vi "Measurement UI.vi"() -> ()   [LabVIEW 2021, in "Line Transient_Channel Ganging UI.lvlib"]
uses:
  Line Transient_Channel Ganging UI.lvlib
panel:
  in  "MeasGraphs":T1(tab)
  out "InputVoltageV/STimeGraph":waveform(dbl)(graph) caption="Load Transient"
  out "OutputVoltageV/STimeGraph":waveform(dbl)(graph) caption="Load Transient"
  in  "Source Voltage v/s Time":string="SOURCE VOLTAGE vs TIME"
  in  "Output Voltage v/s Time":string="LOAD VOLTAGE vs TIME"
  out "InputVoltageV/STimeGraphScope":waveform(dbl)(graph) caption="Load Transient"
  in  "ScopeSource Voltage v/s Time":string="SOURCE VOLTAGE vs TIME"
  out "OutputVoltageV/STimeScope":waveform(dbl)(graph) caption="Load Transient"
  in  "ScopeOutput Voltage v/s Time":string="LOAD VOLTAGE vs TIME"
  out "Scope dt":dbl
  out "Source voltages":dbl[](array[numeric])
  out "Scope amplitudes":dbl[](array[numeric])
  out "Load voltages":dbl[](array[numeric])
  out "Smu dt":dbl
  in  "Load current pole-zero ratio":dbl=0.3
  in  "Load current compensation frequency":dbl=180000.0
  in  "Load current gain bandwidth":dbl=14000.0
  in  "Source voltage pole-zero ratio":dbl=2.0
  in  "Source voltage compensation frequency":dbl=3530.0
  in  "Source voltage gain bandwidth":dbl=2000.0
  in  "Load slave resource names":string[](array[string])
  in  "Load master resource name":string
  in  "Source slave resource names":string[](array[string])
  in  "Source master resource name":string
  in  "Scope resource name":string
  in  "MeasConfigurations":T2(tab)=enum."Source Config"
  in  "Nominal output voltage":dbl=1.0 caption="NOMINAL OUTPUT VOLTAGE" format="%.3pV"
  in  "DUT setup time":dbl=1.0 caption="DUT SETUP TIME" format="%.3ps"
  in  "Source pulse duration":dbl=0.001 caption="PULSE DURATION" format="%.3ps"
  in  "Source time delay 1":dbl=0.001 caption="TIME DELAY 1" format="%.3ps"
  in  "Source time delay 2":dbl=0.001 caption="TIME DELAY 2" format="%.3ps"
  in  "Source voltage level 2":dbl=20.0 caption="VOLTAGE LEVEL 2" format="%#_6pV"
  in  "Source voltage falling slew rate":dbl=6000.0 caption="VOLTAGE FALLING SLEW RATE" format="%#_6pV/s"
  in  "Source voltage rising slew rate":dbl=6000.0 caption="VOLTAGE RISING SLEW RATE" format="%#_6pV/s"
  in  "PPSSlaveResourceNames":refnum<k15>[](array[refnum]) caption="SLAVE RESOURCE NAMES"
  in  "PPSMasterResourceName":refnum<k15> caption="MASTER RESOURCE NAME"
  in  "Source transient response":i32(ring)=1038 caption="TRANSIENT RESPONSE" items=["Slow"=1041, "Normal"=1038, "Fast"=1039, "Custom"=1042]
  in  "Source sense":i32(ring)=1009 caption="SENSE" items=["Local"=1008, "Remote"=1009]
  in  "Source voltage level range":dbl=20.0 caption="VOLTAGE LEVEL RANGE" format="%#_6pV"
  in  "Source voltage level 1":dbl=12.0 caption="VOLTAGE LEVEL 1" format="%#_6pV"
  in  "Source current limit high":dbl=25.0 caption="CURRENT LIMIT/LIMIT HIGH" format="%#_6pA"
  in  "Source current limit range":dbl=25.0 caption="CURRENT LIMIT RANGE" format="%#_6pA"
  in  "Source limit symmetry":enum32{"Symmetric", "Asymmetric"}(ring)=enum."Asymmetric" caption="LIMIT SYMMETRY"
  in  "Source current limit low":dbl=-0.6 caption="CURRENT LIMIT LOW" format="%#_6pA"
  in  "Source system configuration":enum32{"Series", "Parallel"}(ring)=enum."Parallel" caption="SYSTEM CONFIG"
  in  "Source compliance":string="Compliance"
  in  "Source sourceadapt":string="SourceAdapt"
  in  "Source Custom Transient Response":bool
  in  "Source sample rate":dbl=1800000.0 caption="SAMPLE RATE" format="%#_6pS/s"
  in  "Load current level":dbl=1.0 caption="CURRENT LEVEL" format="%#_6pA"
  in  "Load sourceadapt":string="SourceAdapt"
  in  "Load compliance":string="Compliance"
  in  "Load system configuration":enum32{"Series", "Parallel"}(ring)=enum."Parallel" caption="SYSTEM CONFIG"
  in  "Load voltage limit low":dbl caption="VOLTAGE  LIMIT LOW" format="%#_6pV"
  in  "Load limit symmetry":enum32{"Symmetric", "Asymmetric"}(ring) caption="LIMIT SYMMETRY"
  in  "Load voltage limit range":dbl=6.0 caption="VOLTAGE LIMIT RANGE" format="%#_6pV"
  in  "Load voltage limit high":dbl=inf caption="VOLTAGE LIMIT/LIMIT HIGH" format="%#_6p"
  in  "Load current level range":dbl=80.0 caption="CURRENT LEVEL RANGE" format="%#_6pA"
  in  "Load sense":i32(ring)=1009 caption="SENSE" items=["Local"=1008, "Remote"=1009]
  in  "Load transient response":i32(ring)=1038 caption="TRANSIENT RESPONSE" items=["Slow"=1041, "Normal"=1038, "Fast"=1039, "Custom"=1042]
  in  "LoadSlaveResourceNames":refnum<k15>[](array[refnum]) caption="SLAVE RESOURCE NAMES"
  in  "LoadMasterResourceName":refnum<k15> caption="MASTER RESOURCE NAME"
  in  "Load Custom Transient Response":bool
  in  "Scope vertical range":dbl=10.0 caption="VERTICAL RANGE"
  out "Scope status":string="Scope is enabled"
  in  "Scope enable/disable":bool caption="Scope Enable/Disable"
  in  "SCOPEResourceName":refnum<k15> caption="RESOURCE NAME"
  in  "Scope probe attenuation":dbl=1.0 caption="PROBE ATTENUATION"
  in  "Scope sample rate":dbl=1800000.0 caption="SAMPLE RATE" format="%#_6pHz"
  in  "Scope output channel name":string="0" caption="OUTPUT CHANNEL NAME"
  in  "Scope vertical coupling":enum32{"AC", "DC"}(ring)=enum."DC" caption="VERTICAL COUPLING"
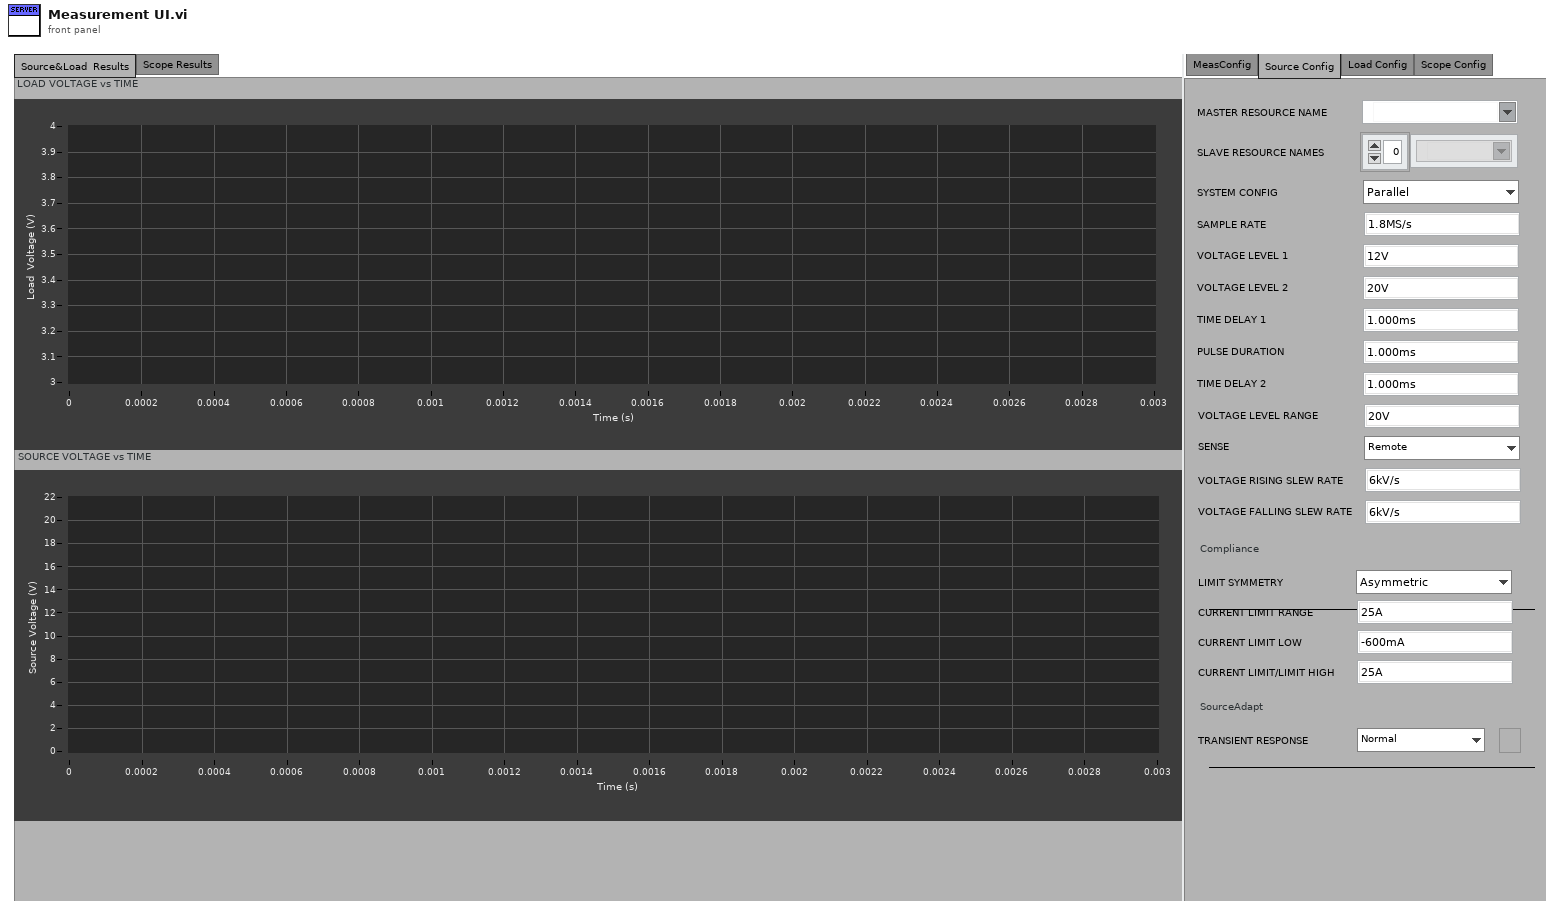
[diagram p1: front panel]
types:
  T1 = enum32{"Source&Load  Results", "Scope Results", "Hidden Controls"}
  T2 = enum32{"MeasConfig", "Source Config", "Load Config", "Scope Config"}
  T3 = typedef "SourceAdapt Parameters.ctl" = cluster{"Voltage gain bandwidth":dbl, "Voltage compensation frequency":dbl, "Voltage pole-zero ratio":dbl, "Current gain bandwidth":dbl, "Current compensation frequency":dbl, "Current pole-zero ratio":dbl}
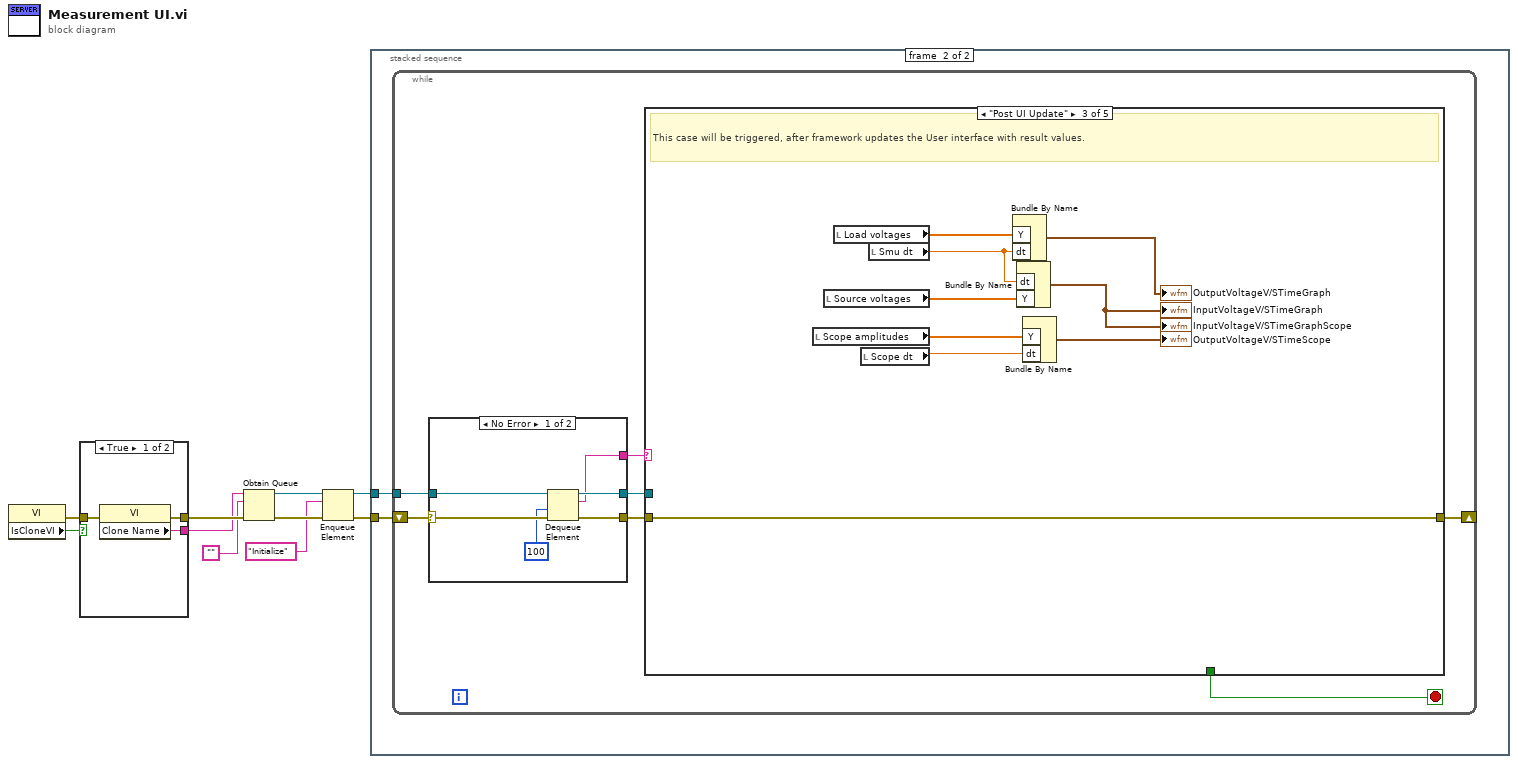
[diagram p0: block diagram]
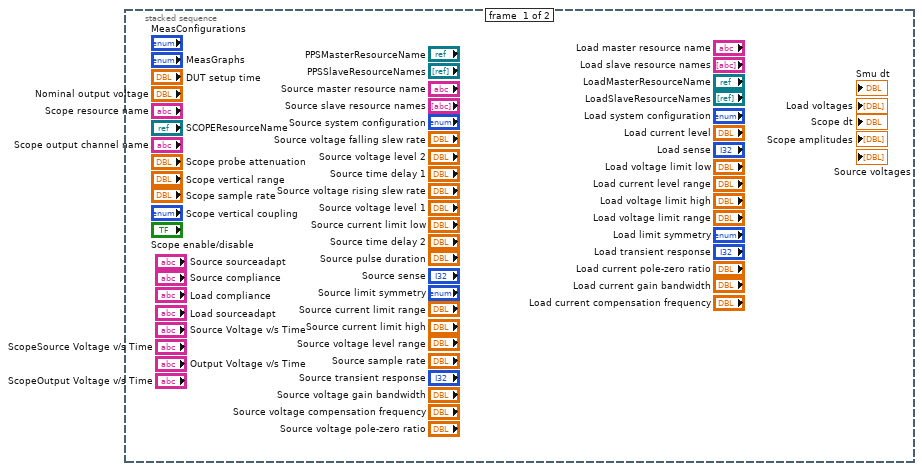
[diagram p2: hidden frame]
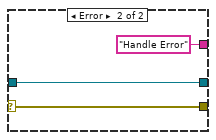
[diagram p3: hidden frame]
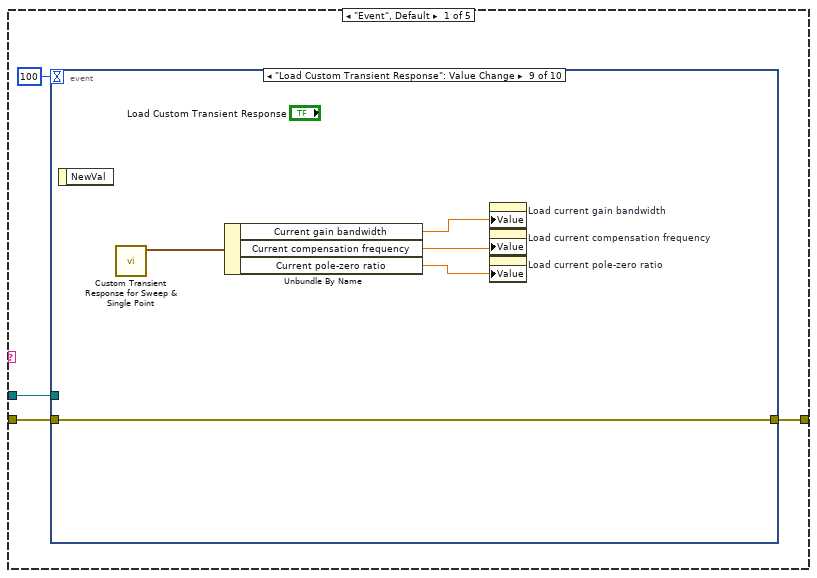
[diagram p4: hidden frame]
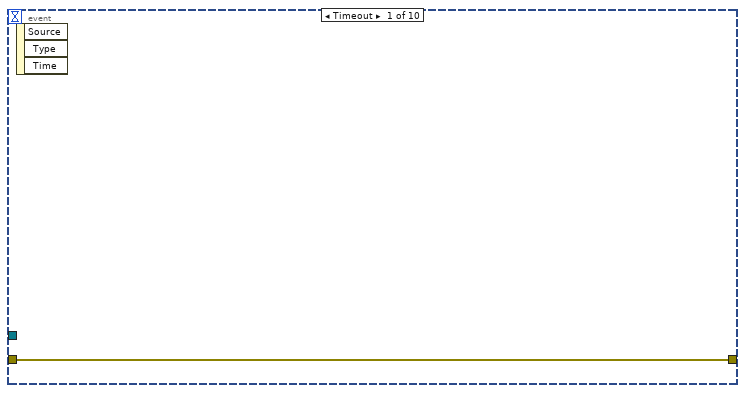
[diagram p5: hidden frame]
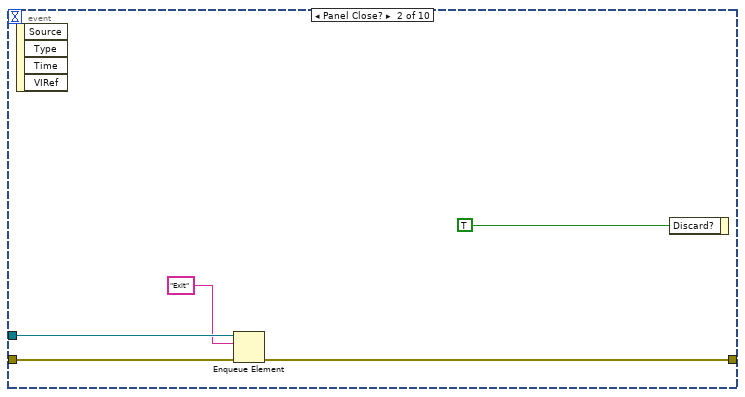
[diagram p6: hidden frame]
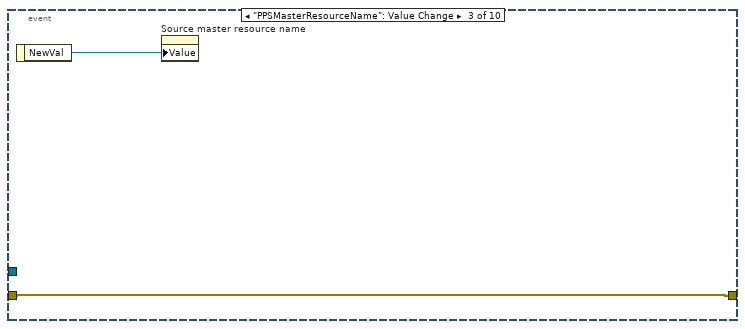
[diagram p7: hidden frame]
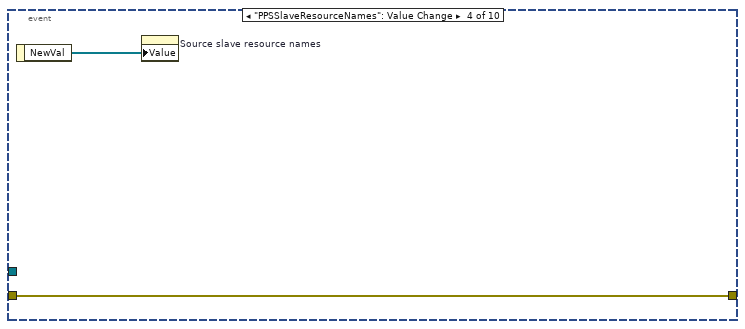
[diagram p8: hidden frame]
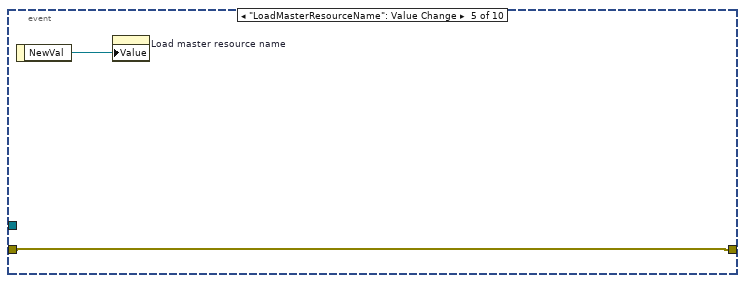
[diagram p9: hidden frame]
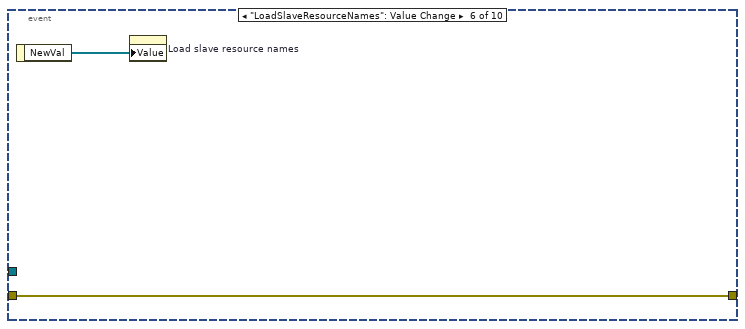
[diagram p10: hidden frame]
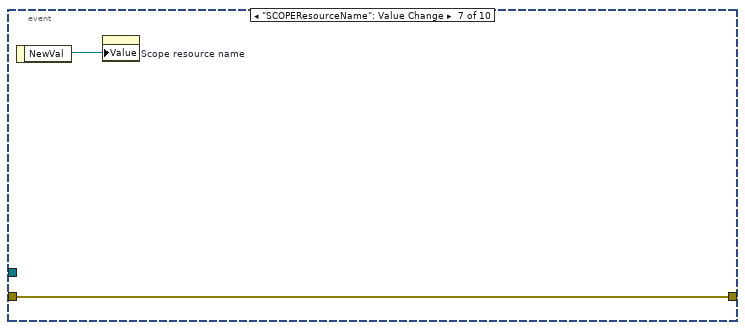
[diagram p11: hidden frame]
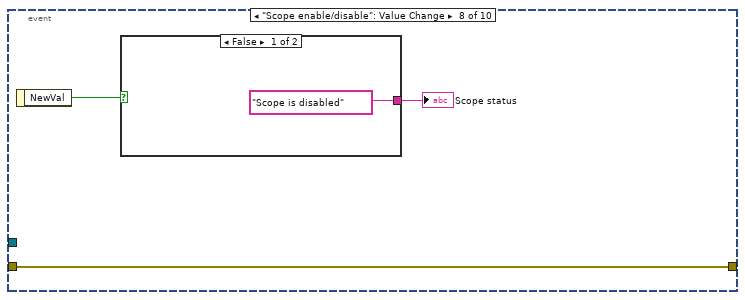
[diagram p12: hidden frame]
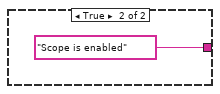
[diagram p13: hidden frame]
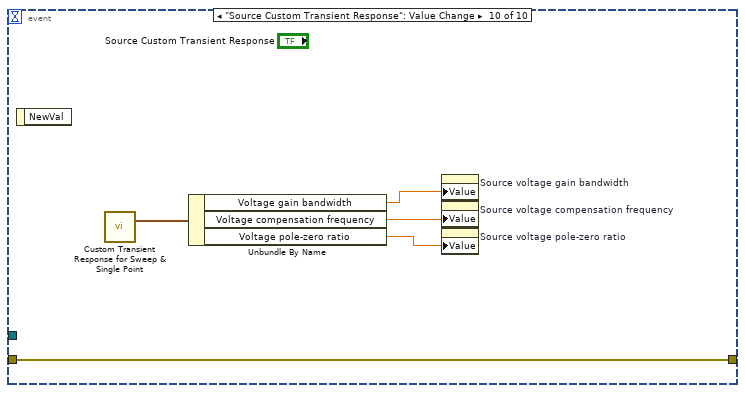
[diagram p14: hidden frame]
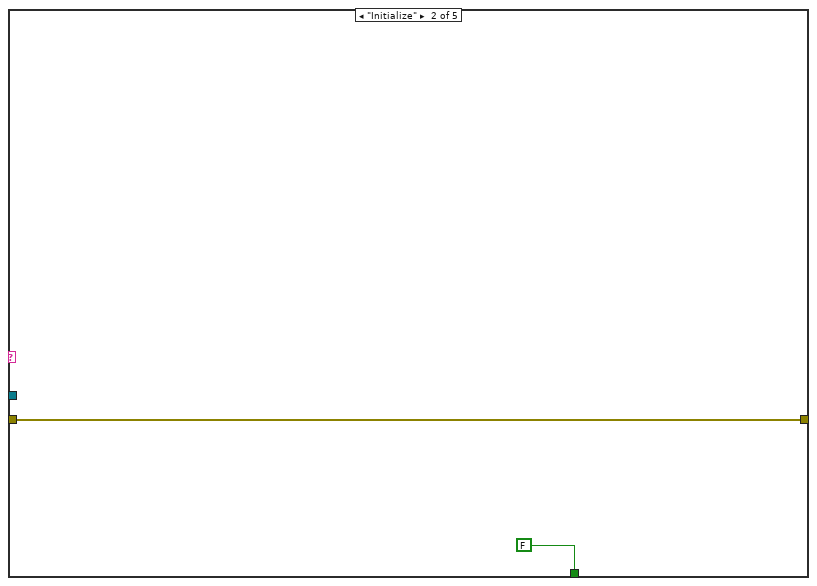
[diagram p15: hidden frame]
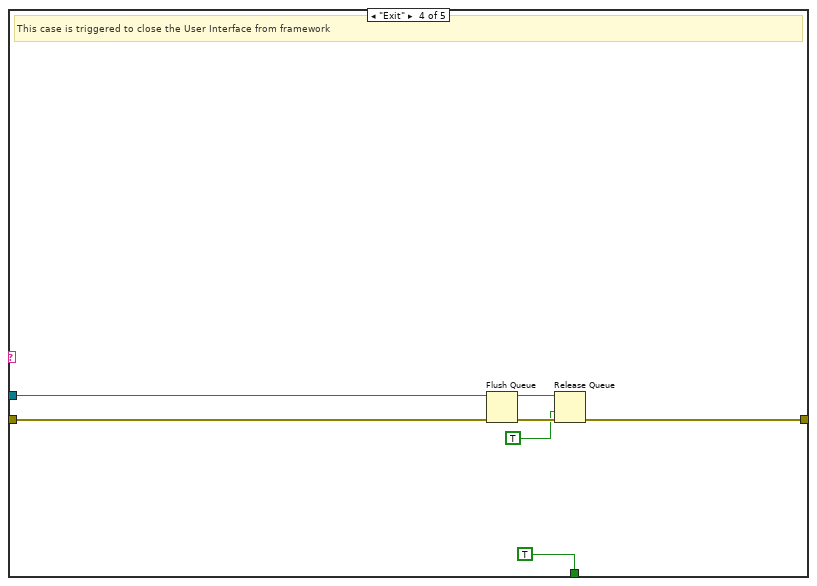
[diagram p16: hidden frame]
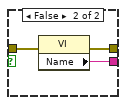
[diagram p18: hidden frame]
diagram:
  n1 = property class="VI"() -> (error out=w1:errorcluster, "IsCloneVI"=w2:bool)  [unwired: 2 in, 1 out]
  n2 = case shown="True" w2 {
    tunnel: [w13 w16] -> w10
    tunnel: [w12 w15] -> w9
    tunnel: w1 -> [w11 w14]
    frame True {
      n3 = property class="VI"(error in=w11) -> (error out=w13:errorcluster, "Clone Name"=w12:string)  [unwired: 1 in, 1 out]
    }
    frame False {
      n4 = property class="VI"(error in=w14) -> (error out=w16:errorcluster, "Name"=w15:string)  [unwired: 1 in, 1 out]
    }
  }
  n5 = Obtain Queue(name (unnamed)=w9, element data type="", error in (no error)=w10) -> (queue out=w6:refnum<queue>, error out=w8:errorcluster)  [unwired: 2 in, 1 out]
  n6 = Enqueue Element(queue=w6, element="Initialize", error in (no error)=w8) -> (queue out=w5:refnum<queue>, error out=w7:errorcluster)  [unwired: 1 in, 1 out]
  n7 = stacked-sequence {
    tunnel: w7 -> [_ w18]
    tunnel: w5 -> [_ w17]
    frame #0 {
    }
    frame #1 {
      n8 = while {
        shift-right: [w20] -> _
        shift-left: w18 -> [w25]
        tunnel: w17 -> [w23]
        stop <- w19 stop-if-true
        n9 = case shown="No Error" w25 {
          selector: w25 -> [w31 w34]
          tunnel: [w30 w34] -> w24
          tunnel: w23 -> [w29 w33]
          tunnel: [w28 w33] -> w22
          tunnel: [w27 "Handle Error"] -> w21
          frame No Error {
            n10 = Dequeue Element(queue=w29, timeout in ms (-1)=100, error in (no error)=w31) -> (queue out=w28:refnum<queue>, element=w27:string, error out=w30:errorcluster)  [unwired: 1 out]
          }
          frame Error {
          }
        }
        n11 = case shown="\"Post UI Update\"" w21 {
          tunnel: w24 -> [w37 w71 w80 w87 w88]
          tunnel: w22 -> [w35 _ _ w85 _]
          tunnel: [w38 w71 w80 w82 w88] -> w20
          tunnel: [_ FALSE _ TRUE _] -> w19
          frame "Event", Default {
            n12 = event shown="[8] \"Load Custom Transient Response\": Value Change" {
              selector: _ -> [_ _ _ _ _ _ _ _ _ _]
              dyn-events: _ -> [_ _ _ _ _ _ _ _ _ _]
              timeout: 100 -> [_ _ _ _ _ _ _ _ _ _]
              tunnel: [w39 w42 w45 w47 w50 w52 w53 w55 w63 w65] -> w38
              tunnel: w37 -> [w39 w43 w45 w47 w50 w52 w53 w55 w63 w65]
              tunnel: w35 -> [_ w41 _ _ _ _ _ _ _ _]
              event Timeout {
                n13 = event-data() -> ()  [unwired: 1 in, 3 out]
              }
              event Panel Close? {
                n14 = event-data() -> ()  [unwired: 1 in, 4 out]
                n15 = Enqueue Element(queue=w41, element="Exit", error in (no error)=w43) -> (error out=w42:errorcluster)  [unwired: 1 in, 2 out]
                n16 = event-data("Discard?"=TRUE) -> ()  [unwired: 1 in, 1 out]
              }
              event "PPSMasterResourceName": Value Change {
                n17 = event-data() -> ("NewVal"=w46:refnum<k15>)  [unwired: 1 in]
                n18 = property on="Source master resource name" class="Str"("Value"=w46) -> ()  [unwired: 2 in, 2 out]
              }
              event "PPSSlaveResourceNames": Value Change {
                n19 = event-data() -> ("NewVal"=w48:refnum<k15>[])  [unwired: 1 in]
                n20 = property on="Source slave resource names" class="Arr (strict)"("Value"=w48) -> ()  [unwired: 2 in, 2 out]
              }
              event "LoadMasterResourceName": Value Change {
                n21 = event-data() -> ("NewVal"=w49:refnum<k15>)  [unwired: 1 in]
                n22 = property on="Load master resource name" class="Str"("Value"=w49) -> ()  [unwired: 2 in, 2 out]
              }
              event "LoadSlaveResourceNames": Value Change {
                n23 = event-data() -> ("NewVal"=w51:refnum<k15>[])  [unwired: 1 in]
                n24 = property on="Load slave resource names" class="Arr (strict)"("Value"=w51) -> ()  [unwired: 2 in, 2 out]
              }
              event "SCOPEResourceName": Value Change {
                n25 = event-data() -> ("NewVal"=w54:refnum<k15>)  [unwired: 1 in]
                n26 = property on="Scope resource name" class="Str"("Value"=w54) -> ()  [unwired: 2 in, 2 out]
              }
              event "Scope enable/disable": Value Change {
                n27 = event-data() -> ("NewVal"=w57:bool)  [unwired: 1 in]
                n28 = case shown="False" w57 {
                  tunnel: ["Scope is disabled" "Scope is enabled"] -> w56
                  frame False {
                  }
                  frame True {
                  }
                }
                "Scope status" <- w56
              }
              event "Load Custom Transient Response": Value Change {
                n29 = event-data() -> ()  [unwired: 1 in, 1 out]
                n30 = call "Custom Transient Response for Sweep & Single Point.vi"() -> ("SourceAdapt Parameters"=w64:T3)  [unwired: 11 in]
                n31 = Unbundle By Name(w64) -> ("Current gain bandwidth"=w60:dbl, "Current compensation frequency"=w62:dbl, "Current pole-zero ratio"=w61:dbl)
                n32 = property on="Load current gain bandwidth" class="DigNum (strict)"("Value"=w60) -> ()  [unwired: 2 in, 2 out]
                n33 = property on="Load current compensation frequency" class="DigNum (strict)"("Value"=w62) -> ()  [unwired: 2 in, 2 out]
                n34 = property on="Load current pole-zero ratio" class="DigNum (strict)"("Value"=w61) -> ()  [unwired: 2 in, 2 out]
              }
              event "Source Custom Transient Response": Value Change {
                n35 = event-data() -> ()  [unwired: 1 in, 1 out]
                n36 = call "Custom Transient Response for Sweep & Single Point.vi"() -> ("SourceAdapt Parameters"=w69:T3)  [unwired: 11 in]
                n37 = Unbundle By Name(w69) -> ("Voltage gain bandwidth"=w68:dbl, "Voltage compensation frequency"=w67:dbl, "Voltage pole-zero ratio"=w66:dbl)
                n38 = property on="Source voltage gain bandwidth" class="DigNum (strict)"("Value"=w68) -> ()  [unwired: 2 in, 2 out]
                n39 = property on="Source voltage compensation frequency" class="DigNum (strict)"("Value"=w67) -> ()  [unwired: 2 in, 2 out]
                n40 = property on="Source voltage pole-zero ratio" class="DigNum (strict)"("Value"=w66) -> ()  [unwired: 2 in, 2 out]
              }
            }
          }
          frame "Initialize" {
          }
          frame "Post UI Update" {
            # "This case will be triggered, after framework updates the User interface with result values."
            n41 = local read "Scope amplitudes"() -> (w76:dbl[])
            n42 = local read "Source voltages"() -> (w78:dbl[])
            n43 = local read "Load voltages"() -> (w79:dbl[])
            n44 = local read "Scope dt"() -> (w75:dbl)
            n45 = local read "Smu dt"() -> (w77:dbl)
            n46 = Bundle By Name("Y"=w79, "dt"=w77) -> (→"OutputVoltageV/STimeGraph":waveform(dbl))  [unwired: 1 in]
            n47 = Bundle By Name("dt"=w77, "Y"=w78) -> (→"InputVoltageV/STimeGraph" →"InputVoltageV/STimeGraphScope":waveform(dbl))  [unwired: 1 in]
            n48 = Bundle By Name("Y"=w76, "dt"=w75) -> (→"OutputVoltageV/STimeScope":waveform(dbl))  [unwired: 1 in]
          }
          frame "Exit" {
            # "This case is triggered to close the User Interface from framework"
            n49 = Flush Queue(queue=w85, error in (no error)=w87) -> (queue out=w84:refnum<queue>, error out=w83:errorcluster)  [unwired: 1 out]
            n50 = Release Queue(queue=w84, force destroy? (F)=TRUE, error in (no error)=w83) -> (error out=w82:errorcluster)  [unwired: 2 out]
          }
          frame "Handle Error" {
          }
        }
      }
    }
  }
